vi "Try To Reconnect.vi"(8 "error in (no error)":errorcluster, 11 "SharedVariableWrapper in":refnum<class "SharedVariableWrapper.lvclass">) -> (0 "error out":errorcluster, 3 "SharedVariableWrapper out":refnum<class "SharedVariableWrapper.lvclass">)   [LabVIEW 2019, in "SharedVariableWrapper.lvclass"]
uses:
  SharedVariableWrapper.lvclass
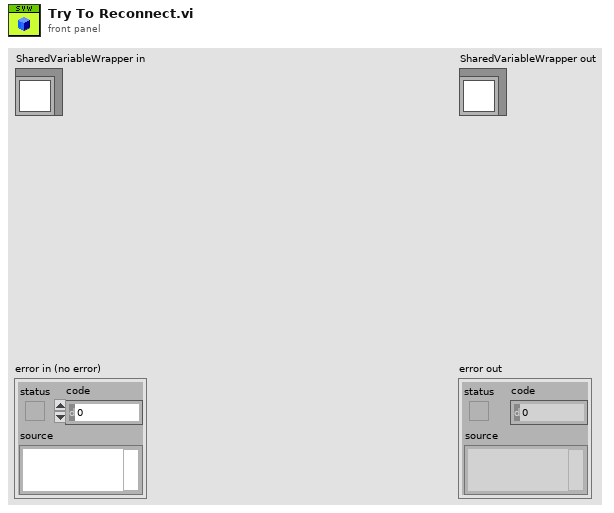
[diagram p1: front panel]
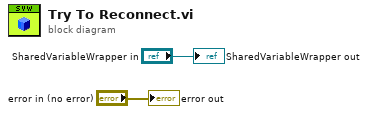
[diagram p0: block diagram]
diagram:
  "error out" <- "error in (no error)"
  "SharedVariableWrapper out" <- "SharedVariableWrapper in"
